vi "Write Zustandsgrössen.Hausmodell.vi"(8 "error in (no error)":errorcluster, 10 "Zustandsgrössen.Hausmodell":T1={"Raumtemperatur [°C]"=15.0, "Bodentemperatur [°C]"=15.0, "Rücklauftemperatur Heizkreislauf [°C]"=15.0}, 11 "Hausmodell in":refnum<class "Hausmodell.lvclass">) -> (0 "error out":errorcluster, 3 "Hausmodell out":refnum<class "Hausmodell.lvclass">)   [LabVIEW 2016, in "Hausmodell.lvclass"]
uses:
  Hausmodell.lvclass
  Hausmodell.lvclass/Hausmodell.ctl
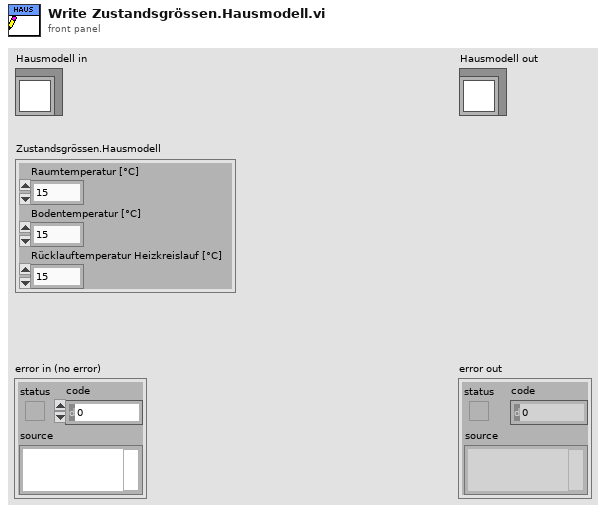
[diagram p1: front panel]
types:
  T1 = typedef "Hausmodell.lvclass/Hausmodell.Zustandsgrössen.ctl" = cluster{"Raumtemperatur [°C]":dbl, "Bodentemperatur [°C]":dbl, "Rücklauftemperatur Heizkreislauf [°C]":dbl}
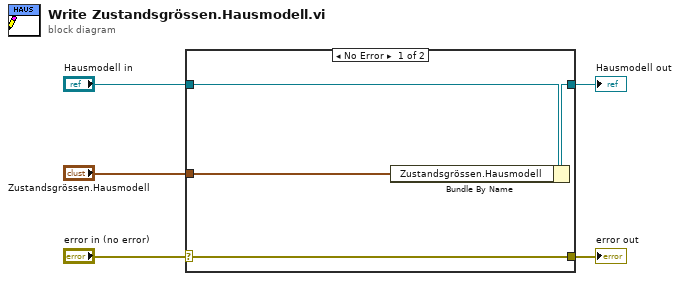
[diagram p0: block diagram]
diagram:
  n1 = case shown="No Error" "error in (no error)" {
    selector: "error in (no error)" -> [w9 w10]
    tunnel: [w9 w10] -> w4
    tunnel: [w7 w11] -> w2
    tunnel: "Hausmodell in" -> [w8 w11]
    tunnel: "Zustandsgrössen.Hausmodell" -> [w6 _]
    frame No Error {
      n2 = Bundle By Name(cluster=w8, "Zustandsgrössen.Hausmodell"=w6) -> (w7:refnum<class "Hausmodell.lvclass">)
    }
    frame Error {
    }
  }
  "error out" <- w4
  "Hausmodell out" <- w2
